vi "statemachine.vi"() -> ()   [LabVIEW 2026]
panel:
  out "State":T1(ring)
  in  "STOP":bool
  in  "Expresso":bool
  in  "Cappuccino":bool
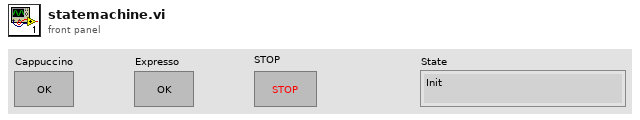
[diagram p1: front panel]
types:
  T1 = enum16{"Init", "Wait", "Cappuccino", "Expresso", "Milk", "Adding Milk", "Release", "Exit", ""}
  T2 = enum16{"Init", "Wait", "Cappuccino", "Expresso", "Milk", "Adding Milk", "Release", "Exit"}
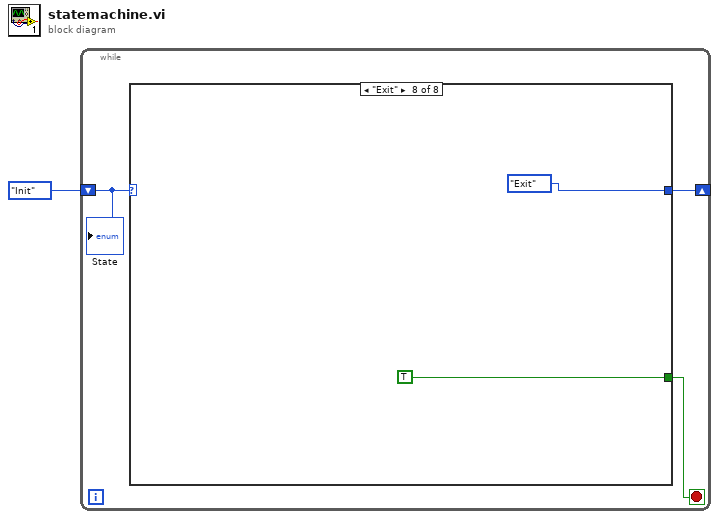
[diagram p0: block diagram]
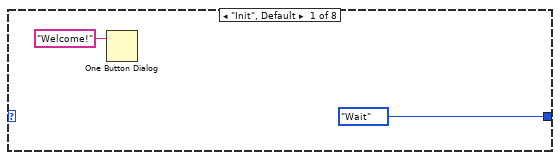
[diagram p2: hidden frame]
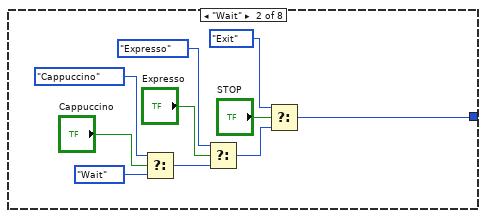
[diagram p3: hidden frame]
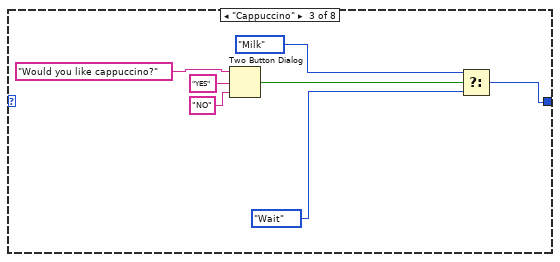
[diagram p4: hidden frame]
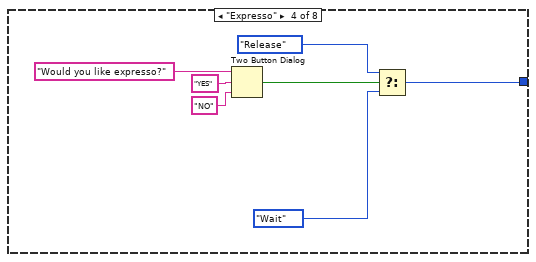
[diagram p5: hidden frame]
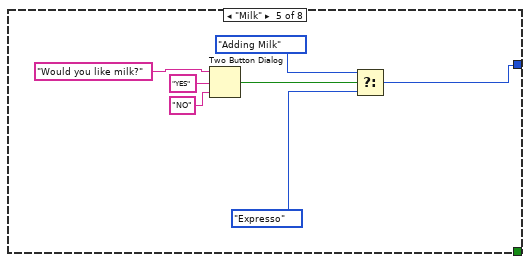
[diagram p6: hidden frame]
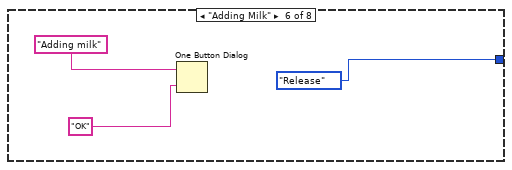
[diagram p7: hidden frame]
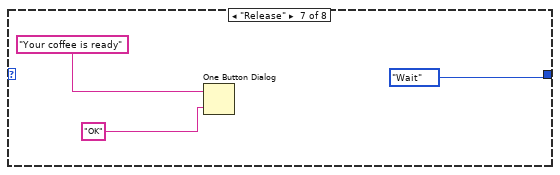
[diagram p8: hidden frame]
diagram:
  n1 = while {
    shift-right: [w4] -> _
    shift-left: T2."Init" -> [w2]
    stop <- w3 stop-if-true
    n2 = case shown="\"Exit\"" w2 {
      tunnel: [T1."Wait" w7 w17 w24 w31 T1."Release" T1."Wait" T1."Exit"] -> w4
      tunnel: [_ _ _ _ _ _ _ TRUE] -> w3
      frame "Init", Default {
        n3 = One Button Dialog(message="Welcome!") -> ()  [unwired: 1 in, 1 out]
      }
      frame "Wait" {
        n4 = Select(t=T1."Cappuccino", s="Cappuccino", f=T1."Wait") -> (s? t:f=w12:T1)
        n5 = Select(t=T1."Expresso", s="Expresso", f=w12) -> (s? t:f=w9:T1)
        n6 = Select(t=T1."Exit", s="STOP", f=w9) -> (s? t:f=w7:T1)
      }
      frame "Cappuccino" {
        n7 = Two Button Dialog(message="Would you like cappuccino?", 1:"NO" ("F button name (\"Cancel\")"), 2:"YES" ("T button name (\"OK\")")) -> (T button?=w23:bool)
        n8 = Select(t=T1."Milk", s=w23, f=T1."Wait") -> (s? t:f=w17:T1)
      }
      frame "Expresso" {
        n9 = Two Button Dialog(message="Would you like expresso?", 1:"NO" ("F button name (\"Cancel\")"), 2:"YES" ("T button name (\"OK\")")) -> (T button?=w27:bool)
        n10 = Select(t=T1."Release", s=w27, f=T1."Wait") -> (s? t:f=w24:T1)
      }
      frame "Milk" {
        n11 = Two Button Dialog(message="Would you like milk?", 1:"NO" ("F button name (\"Cancel\")"), 2:"YES" ("T button name (\"OK\")")) -> (T button?=w37:bool)
        n12 = Select(t=T1."Adding Milk", s=w37, f=T1."Expresso") -> (s? t:f=w31:T1)
      }
      frame "Adding Milk" {
        n13 = One Button Dialog(message="Adding milk", button name ("OK")="OK") -> ()  [unwired: 1 out]
      }
      frame "Release" {
        n14 = One Button Dialog(message="Your coffee is ready", button name ("OK")="OK") -> ()  [unwired: 1 out]
      }
      frame "Exit" {
      }
    }
    "State" <- w2
  }
